vi "Verify Configuration.vi"(0 "eye scan in":refnum<class "niHighSpeedSerial Rectangular Eye Scan v1 Host.lvclass">, 11 "error in":errorcluster) -> (4 "eye scan out":refnum<class "niHighSpeedSerial Rectangular Eye Scan v1 Host.lvclass">, 15 "error out":errorcluster)   [LabVIEW 2014, in "niHighSpeedSerial Rectangular Eye Scan v1 Host.lvclass"]
doc: "Validates that the current configuration is valid before starting Eye Scan on the FPGA.\n\n<B>Input Parameters</B>\n\n<B>eye scan in</B> Takes in a reference to your session from the previous VI.\n\n<B>error in</B> describes error conditions that occur before this node runs. This input provides standard 'error in' functionality.\n\n<B>Output Parameters</B>\n\n<B>eye scan out</B> passes a reference to your session to the next VI.\n\n<B>error out</B> contains error information. This output provides standard 'error out' functionality."
uses:
  <instrlib>/niHighSpeedSerial/Eye Scan/v1/Host/Impl/Rectangular Eye Scan/niHighSpeedSerial Rectangular Eye Scan v1 Host.lvclass
  <instrlib>/niHighSpeedSerial/Eye Scan/v1/Host/Impl/Rectangular Eye Scan/niHighSpeedSerial Rectangular Eye Scan v1 Host.lvclass/niHighSpeedSerial Rectangular Eye Scan v1 Host.ctl
  <vilib>/Utility/error.llb/Error Cluster From Error Code.vi
  <instrlib>/niHighSpeedSerial/Eye Scan/v1/Host/Eye Scan/niHighSpeedSerial Eye Scan v1 Host.lvclass
  <vilib>/ErrorRing/Error Ring.xnode
  <instrlib>/niHighSpeedSerial/Eye Scan/v1/Host/Common/niHighSpeedSerial Eye Scan Common v1 Host.lvlib
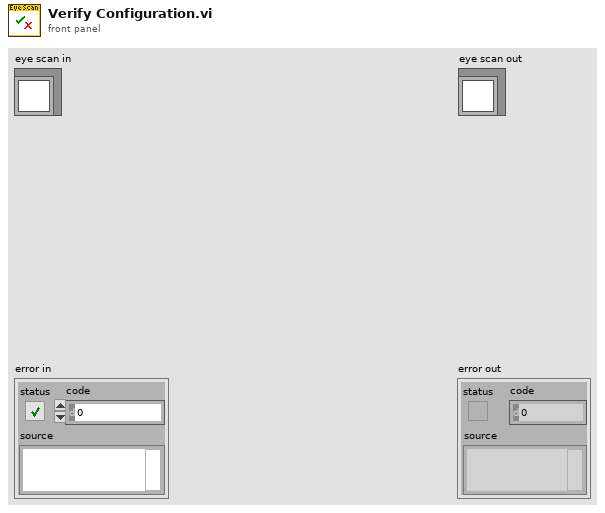
[diagram p1: front panel]
types:
  T1 = typedef "niHighSpeedSerial Eye Scan Common v1 Host.lvlib/RX Output Divider.ctl" = enum16{"1", "2", "4", "8", "16"}
  T2 = typedef "Rectangular Eye Scan v1 Host.lvclass/Private Data.ctl" = cluster{"horizontal step size":i16, "vertical step size":i16, "rectangular eye scan point iterator":refnum<class "niHighSpeedSerial Rectangular Eye Scan Point Iterator v1 Host.lvclass">}
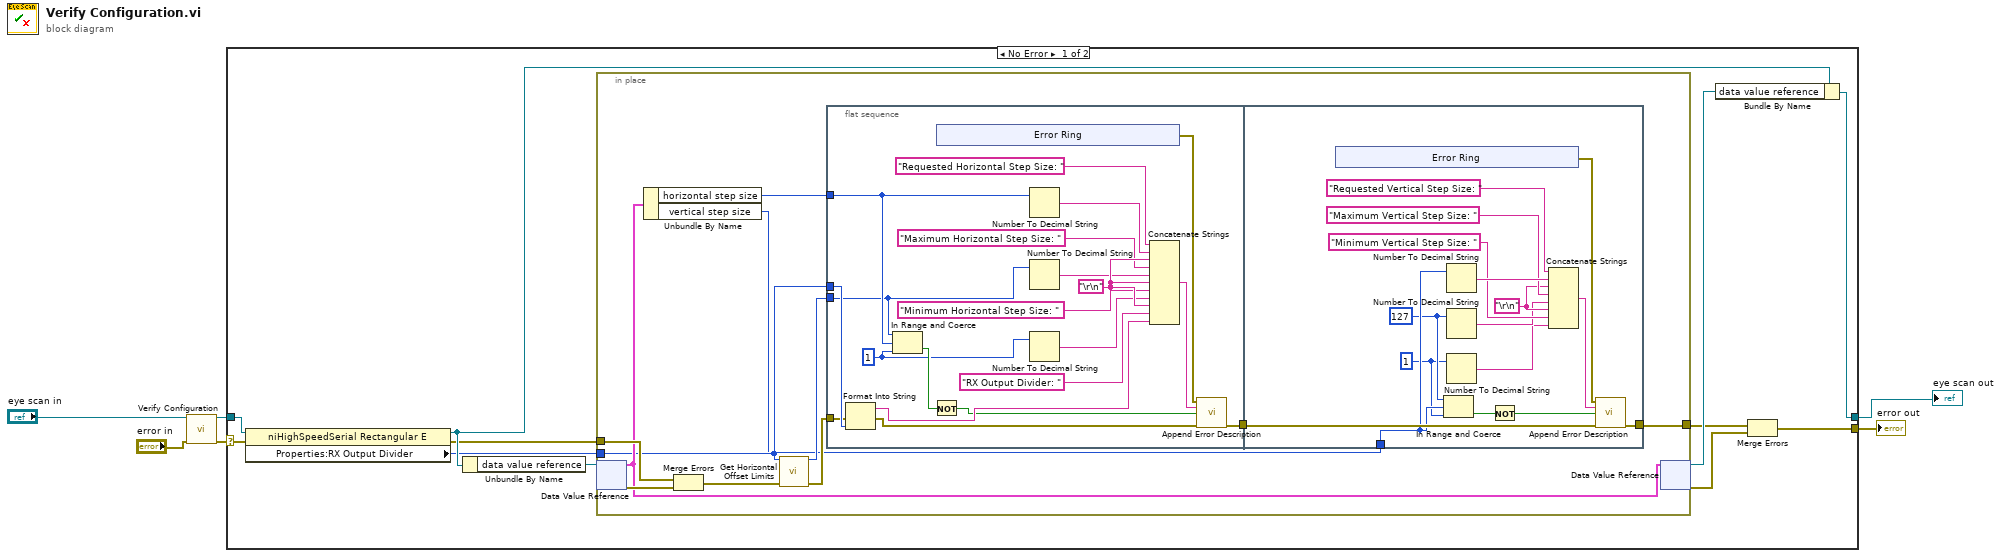
[diagram p0: block diagram]
diagram:
  n1 = call-parent "Verify Configuration.vi"("eye scan in"="eye scan in", "error in"="error in") -> ("eye scan out"=w3:refnum<class "niHighSpeedSerial Rectangular Eye Scan v1 Host.lvclass">, "error out"=w2:errorcluster)  [unwired: 12 in]
  n2 = case shown="No Error" w2 {
    selector: w2 -> [w12 w74]
    tunnel: [w7 w74] -> w6
    tunnel: w3 -> [w14 w73]
    tunnel: [w16 w73] -> w5
    frame No Error {
      n3 = property class="niHighSpeedSerial Rectangular E"(reference=w14, error in=w12) -> (reference out=w13:refnum<class "niHighSpeedSerial Rectangular Eye Scan v1 Host.lvclass">, error out=w10:errorcluster, "Properties:RX Output Divider"=w11:T1)
      n4 = Unbundle By Name(w13) -> ("data value reference"=w17:refnum<data-value>)
      n5 = in-place {
        in-place-border: w11 -> [w21]
        in-place-border: w10 -> [w28]
        in-place-border: [w25] -> w9
        n6 = in-place-dvr #1(w17) -> (w24:T2, w27:errorcluster)
        n7 = Unbundle By Name(w24) -> ("horizontal step size"=w22:i16, "vertical step size"=w18:i16)
        n8 = Merge Errors(w28, w27) -> (w26:errorcluster)
        n9 = call <instrlib>:"Get Horizontal Offset Limits.vi"("rx output divider"=w21, "error in"=w26) -> ("maximum"=w23:i16, "error out"=w20:errorcluster)  [unwired: 10 in, 2 out]
        n10 = flat-sequence {
          tunnel: w23 -> [w29]
          tunnel: w22 -> [w30]
          tunnel: w21 -> [w34]
          tunnel: w20 -> [w33]
          tunnel: [w31] -> w19
          tunnel: [w58] -> w25
          tunnel: w19 -> [w59]
          tunnel: w18 -> [w57]
          frame #0 {
            w35 = i16 1 ("lower limit")
            w48 = "\r\n"
            n11 = Format Into String(error in=w33, w34) -> (resulting string=w47:string, error out=w32:errorcluster)  [unwired: 2 in]
            n12 = In Range and Coerce(upper limit=w29, x=w30, lower limit=w35) -> (In Range?=w36:bool)  [unwired: 1 out]
            n13 = Not(x=w36) -> (.not. x?=w38:bool)
            n14 = xnode "Error Ring"() -> ("error out"=w37:errorcluster)
            n15 = Number To Decimal String(number=w30) -> (decimal integer string=w41:string)  [unwired: 1 in]
            n16 = Number To Decimal String(number=w29) -> (decimal integer string=w43:string)  [unwired: 1 in]
            n17 = Number To Decimal String(number=w35) -> (decimal integer string=w45:string)  [unwired: 1 in]
            n18 = Concatenate Strings("Requested Horizontal Step Size: " ("append string (\"\")"), w41, w48, "Maximum Horizontal Step Size: " ("string"), w43, w48, "Minimum Horizontal Step Size: " ("string"), w45, w48, "RX Output Divider: " ("string"), w47) -> (w40:string)
            n19 = call <instrlib>:"Append Error Description.vi"("error to append"=w37, "append string (\"\")"=w40, "generate error?"=w38, "error in"=w32) -> ("error out"=w31:errorcluster)  [unwired: 11 in]
          }
          frame #1 {
            w61 = "\r\n"
            w54 = i16 1 ("lower limit")
            w56 = i16 127 ("x")
            n20 = xnode "Error Ring"() -> ("error out"=w66:errorcluster)
            n21 = In Range and Coerce(upper limit=w56, x=w57, lower limit=w54) -> (In Range?=w68:bool)  [unwired: 1 out]
            n22 = Number To Decimal String(number=w57) -> (decimal integer string=w64:string)  [unwired: 1 in]
            n23 = Number To Decimal String(number=w56) -> (decimal integer string=w55:string)  [unwired: 1 in]
            n24 = Number To Decimal String(number=w54) -> (decimal integer string=w53:string)  [unwired: 1 in]
            n25 = Not(x=w68) -> (.not. x?=w67:bool)
            n26 = Concatenate Strings("Requested Vertical Step Size: " ("append string (\"\")"), w64, w61, "Maximum Vertical Step Size: " ("string"), w55, w61, "Minimum Vertical Step Size: " ("string"), w53) -> (w63:string)
            n27 = call <instrlib>:"Append Error Description.vi"("error to append"=w66, "append string (\"\")"=w63, "generate error?"=w67, "error in"=w59) -> ("error out"=w58:errorcluster)  [unwired: 11 in]
          }
        }
        n28 = in-place-dvr #1(w24) -> (w15:refnum<data-value>, w8:errorcluster)
      }
      n29 = Bundle By Name(cluster=w13, "data value reference"=w15) -> (w16:refnum<class "niHighSpeedSerial Rectangular Eye Scan v1 Host.lvclass">)
      n30 = Merge Errors(w9, w8) -> (w7:errorcluster)
    }
    frame Error {
    }
  }
  "error out" <- w6
  "eye scan out" <- w5
